vi "Create.vi"(8 "error in (no error)":errorcluster, 11 "MB in":refnum<class "Modbus Master CR.lvclass">) -> (0 "error out":errorcluster, 3 "MB out":refnum<class "Modbus Master CR.lvclass">)   [LabVIEW 2021, in "Modbus Master CR.lvclass"]
uses:
  Modbus Master CR.lvclass
  ctl/MB state.ctl
  ctl/MB_TCP_State.ctl
  Modbus Master CR.lvclass/Modbus Master CR.ctl
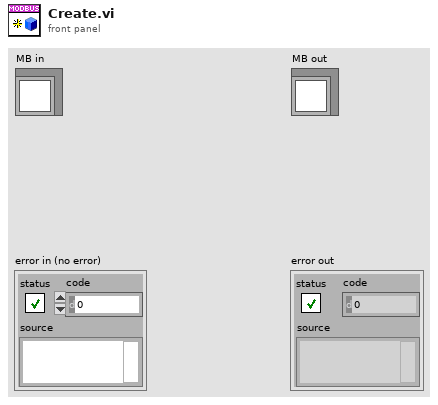
[diagram p1: front panel]
types:
  T1 = typedef "Modbus Master CR.lvclass/MB state.ctl" = cluster{"state":T2, "enable":bool, "Run":bool, "write enable":bool, "Write":bool, "connect":bool, "errors":i32}
  T2 = typedef "Modbus Master CR.lvclass/MB_TCP_State.ctl" = enum8{"initialization", "redefine", "standby", "ping", "connect", "wait to reconnect", "wait to reset timeout", "configure", "requests", "close connection", "stop"}
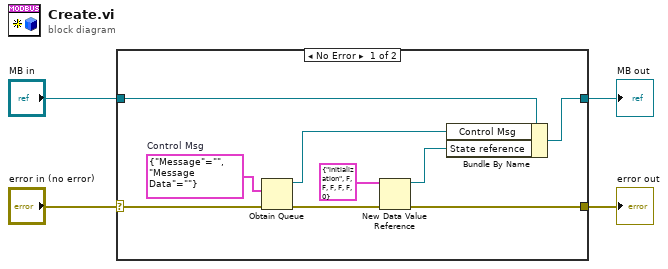
[diagram p0: block diagram]
diagram:
  n1 = case shown="No Error" "error in (no error)" {
    selector: "error in (no error)" -> [w5 w14]
    tunnel: "MB in" -> [w8 w15]
    tunnel: [w7 w14] -> w3
    tunnel: [w6 w15] -> w2
    frame No Error {
      w13 = cluster{"Message":string, "Message Data":string} {"Message"="", "Message Data"=""}  # Control Msg
      n2 = Obtain Queue(element data type=w13, error in (no error)=w5) -> (queue out=w10:refnum<queue>, error out=w9:errorcluster)  [unwired: 3 in, 1 out]
      n3 = New Data Value Reference(data value=T1 {"state"=enum."initialization", "enable"=FALSE, "Run"=FALSE, "write enable"=FALSE, "Write"=FALSE, "connect"=FALSE, "errors"=0} ("State"), error in=w9) -> (data value reference=w11:refnum<data-value>, error out=w7:errorcluster)
      n4 = Bundle By Name(cluster=w8, "Control Msg"=w10, "State reference"=w11) -> (w6:refnum<class "Modbus Master CR.lvclass">)
    }
    frame Error {
    }
  }
  "error out" <- w3
  "MB out" <- w2
